vi "WriteINI.vi"(3 "error in (no error)":errorcluster caption="错误输入（无错误）", 5 "HandsPara":T1={"thumb_servo_max"=136, "thumb_servo_min"=72, "index_servo_max "=146, "index_servo_min"=42, "middle_servo_max "=135, "middle_servo_min"=37, "ring_servo_max"=143, "ring_servo_min"=52, "pinky_servo_max "=143, "pinky_servo_min "=116, "wrist_servo_max"=180, "wrist_servo_min"=0, "arm_servo_max "=84, "arm_servo_min"=15, "rotation_servo_max "=180, "rotation_servo_min "=0}) -> (0 "error out":errorcluster caption="错误输出")   [LabVIEW 2016]
uses:
  Controls/handspara.ctl
  <vilib>/Utility/config.llb/Write Key (U32).vi
  <vilib>/Utility/config.llb/NI_LVConfig.lvlib
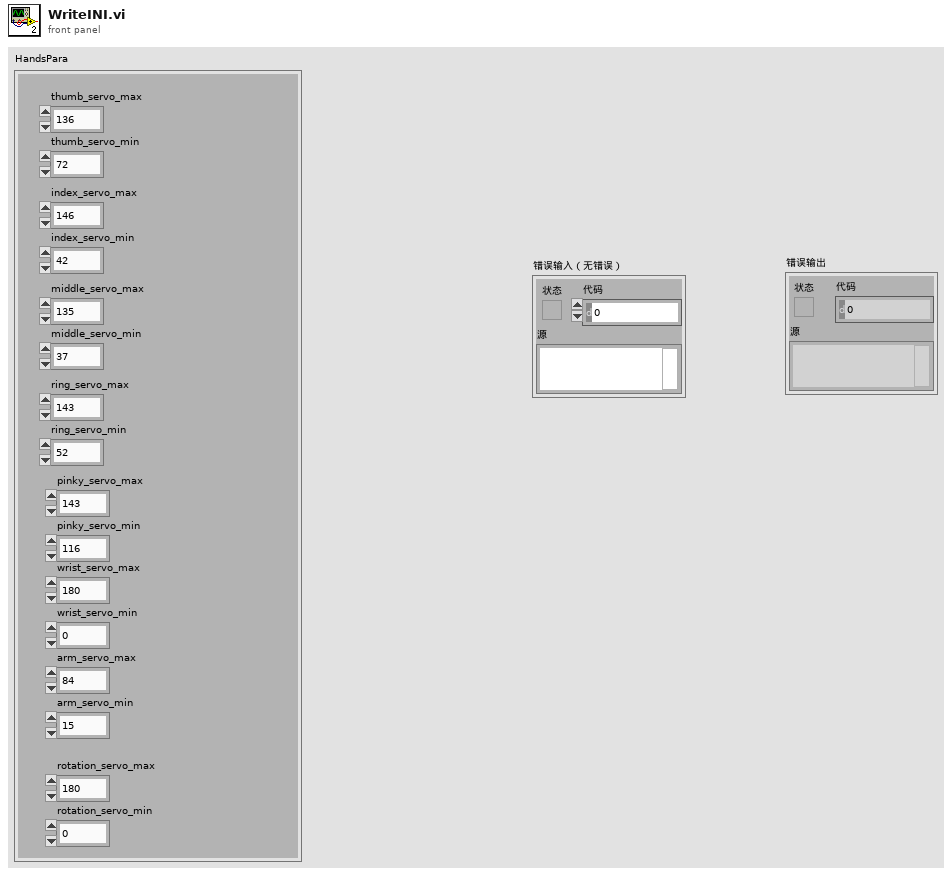
[diagram p1: front panel]
types:
  T1 = typedef "handspara.ctl" = cluster{"thumb_servo_max":u32, "thumb_servo_min":u32, "index_servo_max ":u32, "index_servo_min":u32, "middle_servo_max ":u32, "middle_servo_min":u32, "ring_servo_max":u32, "ring_servo_min":u32, "pinky_servo_max ":u32, "pinky_servo_min ":u32, "wrist_servo_max":u32, "wrist_servo_min":u32, "arm_servo_max ":u32, "arm_servo_min":u32, "rotation_servo_max ":u32, "rotation_servo_min ":u32}
  T2 = typedef "NI_LVConfig.lvlib/Config Data RefNum.ctl" = refnum<k1>
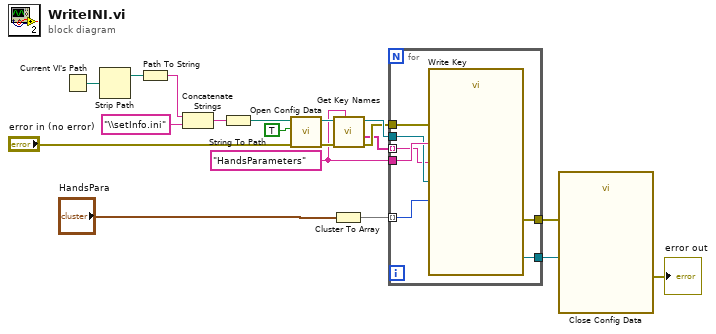
[diagram p0: block diagram]
diagram:
  w3 = "HandsParameters" ("section")
  n1 = Current VI's Path() -> (path=w17:path)
  n2 = Strip Path(path=w17) -> (stripped path=w16:path)  [unwired: 1 out]
  n3 = Path To String(path=w16) -> (string=w19:string)
  n4 = Concatenate Strings(w19, "\\setInfo.ini" ("string")) -> (w18:string)
  n5 = String To Path(string=w18) -> (path=w13:path)
  n6 = call <vilib>:"Open Config Data.vi"("error in (no error)"="error in (no error)", "create file if necessary (T)"=TRUE, "configuration file path"=w13) -> ("error out"=w8:errorcluster, "refnum"=w9:T2)  [unwired: 6 in, 1 out]
  n7 = Cluster To Array(cluster="HandsPara") -> (array=w5:u32[])
  n8 = call <vilib>:"Get Key Names.vi"("section"=w3, "error in (no error)"=w8, "refnum"=w9) -> ("error out"=w6:errorcluster, "key names"=w4:string[], "refnum out"=w7:T2)  [unwired: 5 in, 1 out]
  n9 = for {
    tunnel: w3 -> [w26]
    tunnel: w7 -> [w23]
    tunnel: [w24] -> w10
    tunnel: w6 -> [w22]
    tunnel: [w25] -> w11
    tunnel: w5 -> [w21] mode=indexing
    tunnel: w4 -> [w20] mode=indexing
    n10 = call-poly <vilib>:"Write Key.vi"("section"=w26, "error in (no error)"=w22, "value"=w21, "key"=w20, "refnum"=w23) -> ("error out"=w25:errorcluster, "refnum out"=w24:T2)  [unwired: 4 in, 1 out]
  }
  n11 = call <vilib>:"Close Config Data.vi"("error in (no error)"=w11, "refnum"=w10) -> ("error out"=→"error out":errorcluster)  [unwired: 8 in, 1 out]
